vi "Set Refnums.vi"   [LabVIEW 2014]
uses:
  Global Variables.vi
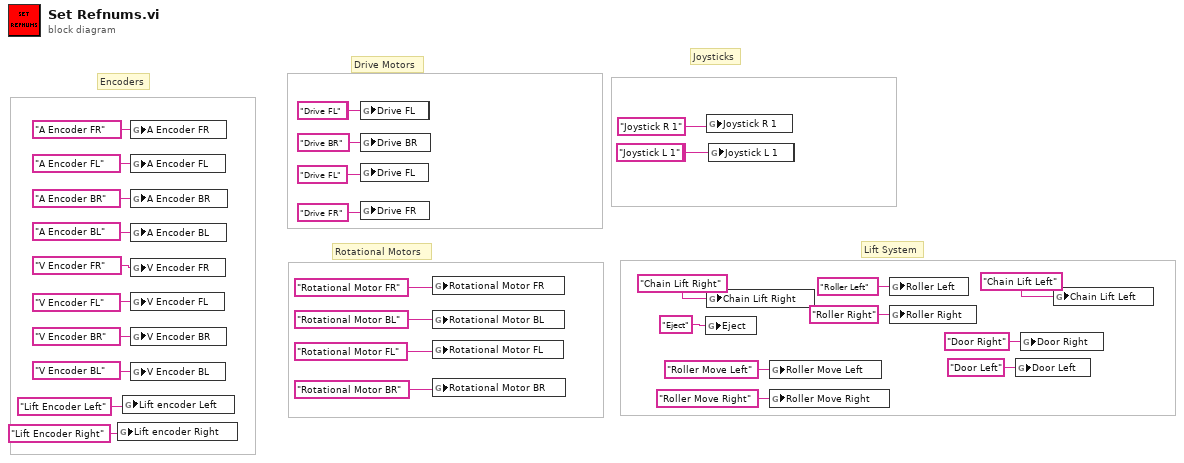
[diagram p0: block diagram]
diagram:
  # "Lift System"
  # "Rotational Motors"
  # "Encoders"
  # "Joysticks"
  # "Drive Motors"
  n1 = global write "Global Variables.vi" "Lift encoder Right"("Lift Encoder Right" ("Lift encoder")) -> ()
  n2 = global write "Global Variables.vi" "Lift encoder Left"("Lift Encoder Left" ("Lift encoder")) -> ()
  n3 = global write "Global Variables.vi" "A Encoder FR"("A Encoder FR") -> ()
  n4 = global write "Global Variables.vi" "A Encoder FL"("A Encoder FL") -> ()
  n5 = global write "Global Variables.vi" "A Encoder BR"("A Encoder BR") -> ()
  n6 = global write "Global Variables.vi" "A Encoder BL"("A Encoder BL") -> ()
  n7 = global write "Global Variables.vi" "V Encoder FR"("V Encoder FR") -> ()
  n8 = global write "Global Variables.vi" "V Encoder FL"("V Encoder FL") -> ()
  n9 = global write "Global Variables.vi" "V Encoder BR"("V Encoder BR") -> ()
  n10 = global write "Global Variables.vi" "V Encoder BL"("V Encoder BL") -> ()
  n11 = global write "Global Variables.vi" "Drive BL"("Drive BL") -> ()
  n12 = global write "Global Variables.vi" "Drive FL"("Drive FL") -> ()
  n13 = global write "Global Variables.vi" "Drive FR"("Drive FR") -> ()
  n14 = global write "Global Variables.vi" "Drive BR"("Drive BR") -> ()
  n15 = global write "Global Variables.vi" "Drive FL"("Drive FL") -> ()
  n16 = global write "Global Variables.vi" "Drive FR"("Drive FR") -> ()
  n17 = global write "Global Variables.vi" "Rotational Motor FR"("Rotational Motor FR") -> ()
  n18 = global write "Global Variables.vi" "Rotational Motor BL"("Rotational Motor BL") -> ()
  n19 = global write "Global Variables.vi" "Rotational Motor FL"("Rotational Motor FL") -> ()
  n20 = global write "Global Variables.vi" "Rotational Motor BR"("Rotational Motor BR") -> ()
  n21 = global write "Global Variables.vi" "Eject"("Eject") -> ()
  n22 = global write "Global Variables.vi" "Joystick R 1"("Joystick R 1" ("Joystick R 1")) -> ()
  n23 = global write "Global Variables.vi" "Chain Lift Right"("Chain Lift Right") -> ()
  n24 = global write "Global Variables.vi" "Joystick L 1"("Joystick L 1" ("Joystick R 1")) -> ()
  n25 = global write "Global Variables.vi" "Joystick R 1"("Joystick R 1" ("Joystick R 1")) -> ()
  n26 = global write "Global Variables.vi" "Roller Move Left"("Roller Move Left") -> ()
  n27 = global write "Global Variables.vi" "Roller Move Right"("Roller Move Right") -> ()
  n28 = global write "Global Variables.vi" "Roller Left"("Roller Left") -> ()
  n29 = global write "Global Variables.vi" "Roller Right"("Roller Right") -> ()
  n30 = global write "Global Variables.vi" "Door Left"("Door Left") -> ()
  n31 = global write "Global Variables.vi" "Door Right"("Door Right") -> ()
  n32 = global write "Global Variables.vi" "Chain Lift Left"("Chain Lift Left") -> ()
